vi "reorder modules based on execution order.vi"(8 "error in":errorcluster, 9 "module configs":refnum<class "TBM module configuration.lvclass">[](array[class]), 10 "module runtimes":refnum<class "TBM module execution interface.lvclass">[](array[class]), 11 "Standard Engine Configuration":refnum<class "Standard Engine Configuration.lvclass">) -> (0 "error out":errorcluster, 1 "module configs out":refnum<class "TBM module configuration.lvclass">[](array[class]), 2 "module runtimes out":refnum<class "TBM module execution interface.lvclass">[](array[class]), 3 "Standard Engine Configuration Out":refnum<class "Standard Engine Configuration.lvclass">)   [LabVIEW 2013, in "Standard Engine Runtime.lvclass"]
doc: "Reorders the modules in the runtime and config arrays based on the execution order specified in the standard engine config.\n\nThis VI assumes that the module runtimes and module configs arrays are the same size and contain modules in the same order."
uses:
  Standard Engine Runtime.lvclass
  <vilib>/NI/Tag Bus Module Framework/runtime/TBM module execution interface.lvclass
  Configuration/Standard Engine Configuration.lvclass
  <vilib>/NI/Tag Bus Module Framework/module configuration/TBM module configuration.lvclass
  <vilib>/NI/Configuration Framework/serializable configuration/NISE_CEF_serializable configuration.lvclass/NISE_CEF_serializable configuration.ctl
  Configuration/Standard Engine Configuration.lvclass/Standard Engine Configuration.ctl
  <vilib>/Utility/LVClass/Get LV Class Name.vi
  <vilib>/NI/Configuration Framework/error generator/NISE_error generator.vi
  Configuration/Find Module Specific Config.vi
  <vilib>/NI/Configuration Framework/serializable configuration/NISE_CEF_serializable configuration.lvclass
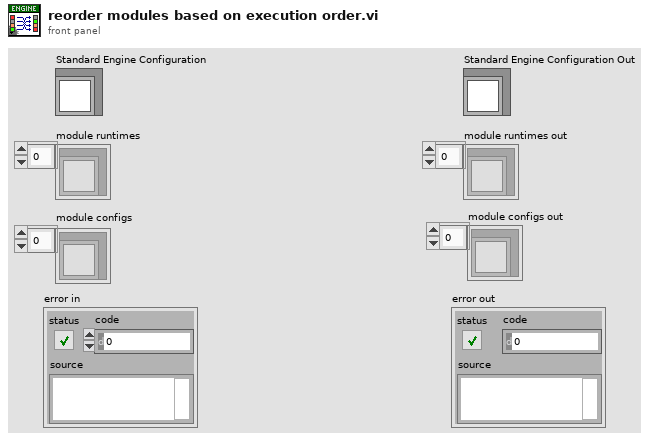
[diagram p1: front panel]
types:
  T1 = cluster{"execution order priority":i32, "Component Runtime Interface.lvclass":refnum<class "TBM module execution interface.lvclass">, "configuration out":refnum<class "TBM module configuration.lvclass">}
  T2 = cluster{"execution order priority":i32, "Component Runtime Interface.lvclass":refnum<class "TBM module execution interface.lvclass">, "configuration out":refnum<class "TBM module configuration.lvclass">}[]
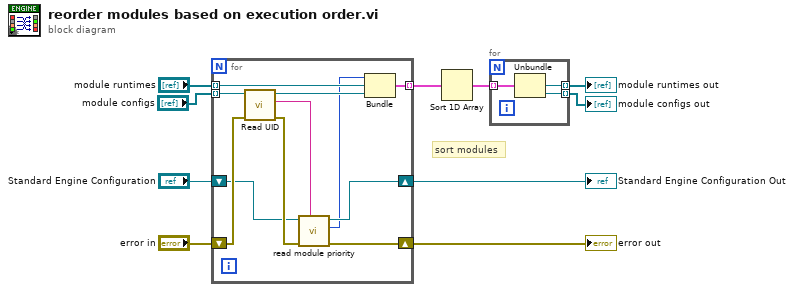
[diagram p0: block diagram]
diagram:
  # "sort modules"
  n1 = for {
    tunnel: "module configs" -> [w21] mode=indexing
    shift-right: [w17] -> w3
    shift-left: "Standard Engine Configuration" -> [w15]
    tunnel: "module runtimes" -> [w14] mode=indexing
    shift-right: [w20] -> w2
    shift-left: "error in" -> [w19]
    tunnel: [w11] -> w10 mode=indexing
    n2 = call <vilib>:"Read UID.vi"("error in"=w19, "configuration in"=w21) -> ("error out"=w18:errorcluster, "instance id"=w16:string, "configuration out"=w13:refnum<class "TBM module configuration.lvclass">)  [unwired: 7 in]
    n3 = call "read module priority.vi"("Module ID"=w16, "error in"=w18, "Standard Engine Repo Data in"=w15) -> ("error out"=w20:errorcluster, "execution order priority"=w12:i32, "Standard Engine Repo Data out"=w17:refnum<class "Standard Engine Configuration.lvclass">)  [unwired: 6 in]
    n4 = Bundle("execution order priority"=w12, "Component Runtime Interface.lvclass"=w14, "configuration out"=w13) -> (w11:T1)  [unwired: 1 in]
  }
  "Standard Engine Configuration Out" <- w3
  "error out" <- w2
  n5 = Sort 1D Array(array=w10) -> (sorted array=w9:T2)
  n6 = for {
    tunnel: w9 -> [w24] mode=indexing
    tunnel: [w23] -> w5 mode=indexing
    tunnel: [w22] -> w4 mode=indexing
    n7 = Unbundle(w24) -> ("Component Runtime Interface.lvclass"=w23:refnum<class "TBM module execution interface.lvclass">, "configuration out"=w22:refnum<class "TBM module configuration.lvclass">)  [unwired: 1 out]
  }
  "module runtimes out" <- w5
  "module configs out" <- w4
